vi "Set All Active UUTs to Testing.vi"(8 "error in (no error)":errorcluster, 11 "Application in":refnum<class "Application.lvclass">) -> (0 "error out":errorcluster, 2 "Number of Active DUTs":i32, 3 "Application out":refnum<class "Application.lvclass">)   [LabVIEW 2017, in "Application.lvlib" / "Application.lvclass"]
doc: "Updates the State of all UUTs in the Ready state to Testing. Typically used when starting a test."
uses:
  Application.lvclass
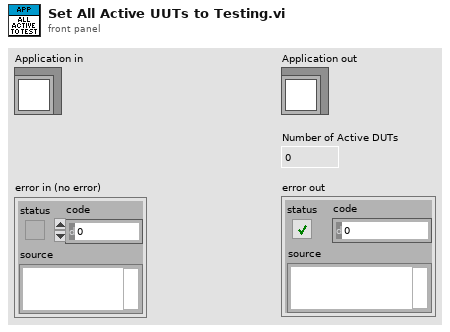
[diagram p1: front panel]
types:
  T1 = cluster{"Serial Number Reference":refnum<vi>, "Status Message Reference":refnum<vi>, "Position":u32}[]
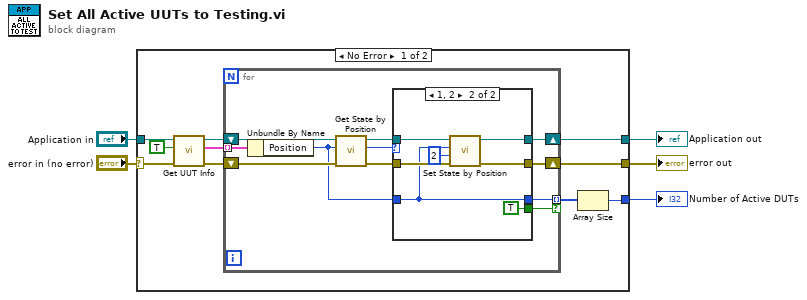
[diagram p0: block diagram]
diagram:
  n1 = case shown="No Error" "error in (no error)" {
    selector: "error in (no error)" -> [w7 w37]
    tunnel: [w15 w38] -> w5
    tunnel: "Application in" -> [w11 w38]
    tunnel: [w14 w37] -> w2
    tunnel: [w12 _] -> w1
    frame No Error {
      n2 = call-dynamic "Get UUT Info.vi"("error in (no error)"=w7, "Scanned Only (false)"=TRUE, "Application in"=w11) -> ("error out"=w9:errorcluster, "All UUTs"=w8:T1, "Application out"=w10:refnum<class "Application.lvclass">)  [unwired: 6 in]
      n3 = for {
        shift-right: [w26] -> w15
        shift-left: w10 -> [w24]
        tunnel: w8 -> [w25] mode=indexing
        shift-right: [w20] -> w14
        shift-left: w9 -> [w21]
        tunnel: [w17] -> w13 mode=indexing if=w16
        n4 = Unbundle By Name(w25) -> ("Position"=w18:u32)
        n5 = call-dynamic "Get State by Position.vi"("error in (no error)"=w21, "Position"=w18, "Application in"=w24) -> ("error out"=w19:errorcluster, "State"=w22:u32, "Application out"=w23:refnum<class "Application.lvclass">)  [unwired: 6 in]
        n6 = case shown="1, 2" w22 {
          tunnel: [w29 w35] -> w26
          tunnel: w23 -> [w29 w36]
          tunnel: [w28 w34] -> w20
          tunnel: w19 -> [w28 w33]
          tunnel: w18 -> [w27 w31]
          tunnel: [w27 w31] -> w17
          tunnel: [_ TRUE] -> w16
          frame 0, Default {
          }
          frame 1, 2 {
            n7 = call-dynamic "Set State by Position.vi"("error in (no error)"=w33, "State"=u32 2, "Position"=w31, "Application in"=w36) -> ("error out"=w34:errorcluster, "Application out"=w35:refnum<class "Application.lvclass">)  [unwired: 6 in]
          }
        }
      }
      n8 = Array Size(array=w13) -> (size(s)=w12:i32)
    }
    frame Error {
    }
  }
  "Application out" <- w5
  "error out" <- w2
  "Number of Active DUTs" <- w1
